vi "contador.vi"() -> ()   [LabVIEW 2009]
panel:
  out "y":dbl
  out "?":u8
  out "decimal integer string":string
  out "floor(x/y)":i32
  out "array":dbl[][](array[numeric])
  out "Array":dbl[][][](array[numeric])
  out "data out":string
  in  "id":i32
  in  "buffer":i32=300
  in  "number data":i32=1
  out "adreça":i32
  in  "command":i32
  in  "stop":bool
  in  "Send":bool
  out "data logged":string
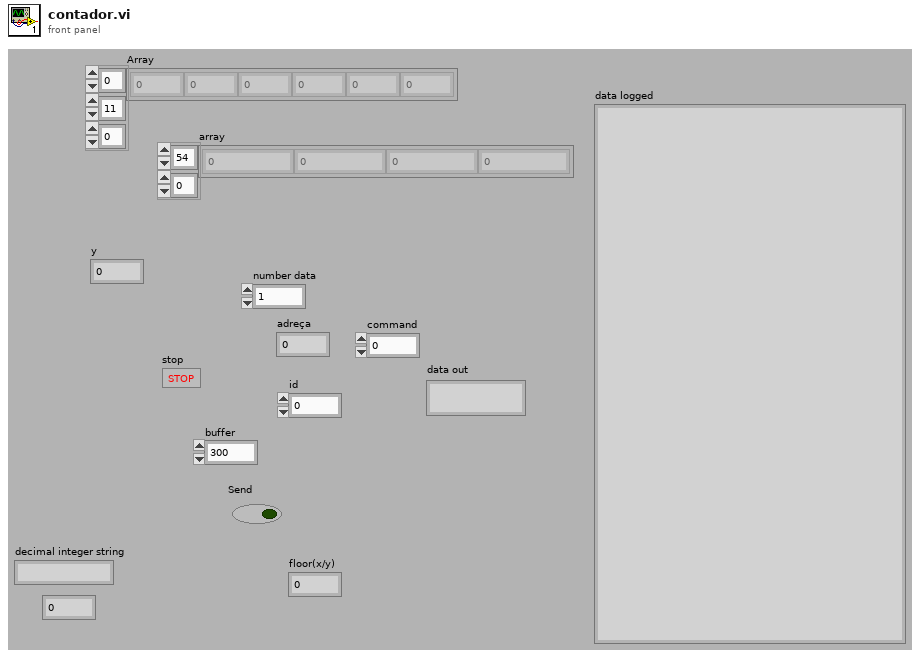
[diagram p1: front panel]
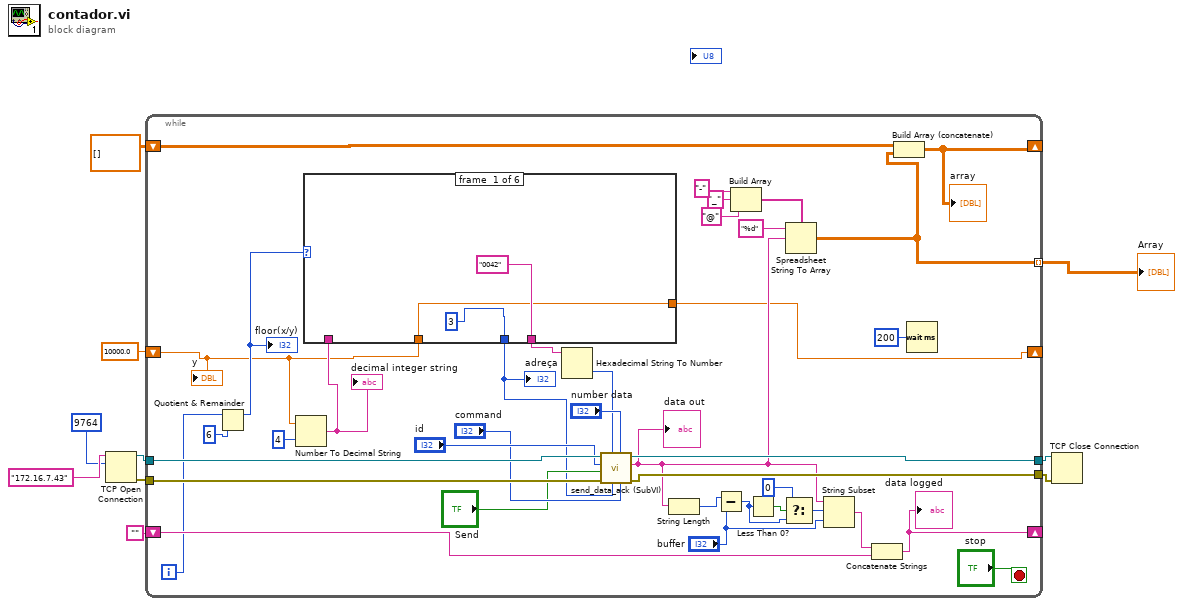
[diagram p0: block diagram]
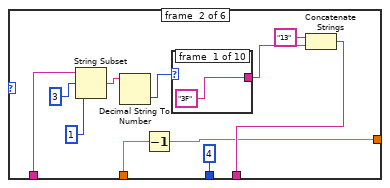
[diagram p2: hidden frame]
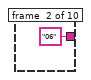
[diagram p3: hidden frame]
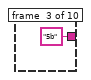
[diagram p4: hidden frame]
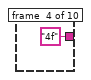
[diagram p5: hidden frame]
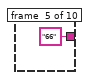
[diagram p6: hidden frame]
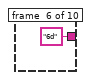
[diagram p7: hidden frame]
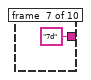
[diagram p8: hidden frame]
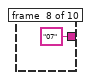
[diagram p9: hidden frame]
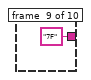
[diagram p10: hidden frame]
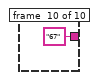
[diagram p11: hidden frame]
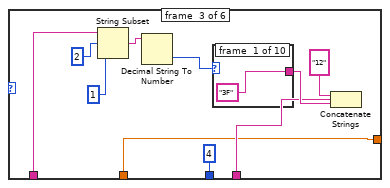
[diagram p12: hidden frame]
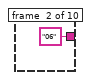
[diagram p13: hidden frame]
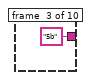
[diagram p14: hidden frame]
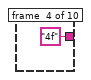
[diagram p15: hidden frame]
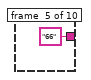
[diagram p16: hidden frame]
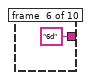
[diagram p17: hidden frame]
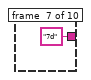
[diagram p18: hidden frame]
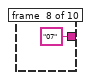
[diagram p19: hidden frame]
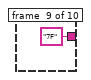
[diagram p20: hidden frame]
diagram:
  n1 = TCP Open Connection(address="172.16.7.43", remote port or service name=u16 9764) -> (connection ID=w5:refnum<k5>, error out=w4:errorcluster)  [unwired: 3 in]
  n2 = while {
    shift-right: [w40] -> _
    shift-left: "" -> [w39]
    tunnel: [w38] -> w9
    tunnel: [w37] -> w8
    tunnel: w5 -> [w36]
    tunnel: w4 -> [w35]
    tunnel: [w25] -> w3 mode=indexing
    shift-right: [w23] -> _
    shift-left: dbl[][] [] -> [w24]
    shift-right: [w12] -> _
    shift-left: 10000.0 ("y") -> [w11]
    i -> [w13]
    stop <- "stop" stop-if-true
    n3 = Quotient & Remainder(x=w13, y=6) -> (x-y*floor(x/y)=w16:i32)  [unwired: 1 out]
    "floor(x/y)" <- w16
    n4 = Number To Decimal String(number=w11, width (-)=i16 4) -> (decimal integer string=w14:string)
    "decimal integer string" <- w14
    n5 = case shown="3" w16 {
      tunnel: [3 ("adreça") 4 ("adreça") 4 ("adreça") 3 ("adreça") 4 ("adreça") 4 ("adreça")] -> w18
      tunnel: ["0042" ("string") w60 w79 "0040" ("string") w103 w122] -> w19
      tunnel: w14 -> [_ w58 w74 _ w97 w118]
      tunnel: w11 -> [w49 w53 w73 w93 w96 w116]
      tunnel: [w49 w52 w73 w93 w96 w116] -> w12
      frame #0 {
      }
      frame #1 {
        n6 = String Subset(string=w58, offset (0)=3 ("index"), length (rest)=1 ("length (rest)")) -> (substring=w55:string)
        n7 = Decimal String To Number(string=w55) -> (number=w54:i32)  [unwired: 2 in, 1 out]
        n8 = Decrement(x=w53) -> (x-1=w52:dbl)
        n9 = case shown="5" w54 {
          tunnel: ["3F" ("Data hex") "06" ("Data hex") "5b" ("Data hex") "4f" ("Data hex") "66" ("Data hex") "6d" ("Data hex") "7d" ("Data hex") "07" ("Data hex") "7F" ("Data hex") "67" ("Data hex")] -> w62
          frame #0 {
          }
          frame #1 {
          }
          frame #2 {
          }
          frame #3 {
          }
          frame #4 {
          }
          frame #5 {
          }
          frame #6 {
          }
          frame #7 {
          }
          frame #8 {
          }
          frame #9 {
          }
        }
        n10 = Concatenate Strings("13" ("string"), w62) -> (w60:string)
      }
      frame #2 {
        n11 = String Subset(string=w74, offset (0)=2 ("index"), length (rest)=1 ("length (rest)")) -> (substring=w76:string)
        n12 = Decimal String To Number(string=w76) -> (number=w75:i32)  [unwired: 2 in, 1 out]
        n13 = case shown="5" w75 {
          tunnel: ["3F" ("Data hex") "06" ("Data hex") "5b" ("Data hex") "4f" ("Data hex") "66" ("Data hex") "6d" ("Data hex") "7d" ("Data hex") "07" ("Data hex") "7F" ("Data hex") "67" ("Data hex")] -> w82
          frame #0 {
          }
          frame #1 {
          }
          frame #2 {
          }
          frame #3 {
          }
          frame #4 {
          }
          frame #5 {
          }
          frame #6 {
          }
          frame #7 {
          }
          frame #8 {
          }
          frame #9 {
          }
        }
        n14 = Concatenate Strings("12" ("string"), w82) -> (w79:string)
      }
      frame #3 {
      }
      frame #4 {
        n15 = String Subset(string=w97, offset (0)=1 ("index"), length (rest)=1 ("length (rest)")) -> (substring=w99:string)
        n16 = Decimal String To Number(string=w99) -> (number=w98:i32)  [unwired: 2 in, 1 out]
        n17 = case shown="9" w98 {
          tunnel: ["3F" ("Data hex") "06" ("Data hex") "5b" ("Data hex") "4f" ("Data hex") "66" ("Data hex") "6d" ("Data hex") "7d" ("Data hex") "07" ("Data hex") "7F" ("Data hex") "67" ("Data hex")] -> w105
          frame #0 {
          }
          frame #1 {
          }
          frame #2 {
          }
          frame #3 {
          }
          frame #4 {
          }
          frame #5 {
          }
          frame #6 {
          }
          frame #7 {
          }
          frame #8 {
          }
          frame #9 {
          }
        }
        n18 = Concatenate Strings("13" ("string"), w105) -> (w103:string)
      }
      frame #5 {
        n19 = String Subset(string=w118, offset (0)=0 ("index"), length (rest)=1 ("length (rest)")) -> (substring=w120:string)
        n20 = Decimal String To Number(string=w120) -> (number=w119:i32)  [unwired: 2 in, 1 out]
        n21 = case shown="5" w119 {
          tunnel: ["3F" ("Data hex") "06" ("Data hex") "5b" ("Data hex") "4f" ("Data hex") "66" ("Data hex") "6d" ("Data hex") "7d" ("Data hex") "07" ("Data hex") "7F" ("Data hex") "67" ("Data hex")] -> w125
          frame #0 {
          }
          frame #1 {
          }
          frame #2 {
          }
          frame #3 {
          }
          frame #4 {
          }
          frame #5 {
          }
          frame #6 {
          }
          frame #7 {
          }
          frame #8 {
          }
          frame #9 {
          }
        }
        n22 = Concatenate Strings("12" ("string"), w125) -> (w122:string)
      }
    }
    "adreça" <- w18
    n23 = Hexadecimal String To Number(string=w19) -> (number=w20:u32)  [unwired: 2 in, 1 out]
    n24 = call "send_data_ack (SubVI).vi"("command"="command", "number data"="number data", "adreça"=w18, "Dada"=w20, "error out"=w35, "Send"="Send", "id"="id", "connection ID"=w36) -> ("error out 2"=w37:errorcluster, "data out"=w31:string, "connection ID out"=w38:refnum<k5>)  [unwired: 1 out]
    "data out" <- w31
    n25 = String Length(string=w31) -> (length=w47:i32)
    n26 = Subtract(x=w47, y="buffer") -> (x-y=w44:i32)
    n27 = Build Array("-" ("spreadsheet string"), "_" ("element"), "@" ("element")) -> (w29:string[])
    n28 = Less Than 0?(x=w44) -> (x < 0?=w46:bool)
    n29 = Select(t=0, s=w46, f=w44) -> (s? t:f=w43:i32)
    n30 = Spreadsheet String To Array(delimiter (Tab)=w29, format string="%d", spreadsheet string=w31) -> (array=w25:dbl[][])  [unwired: 1 in]
    n31 = String Subset(string=w31, offset (0)=w43, length (rest)="buffer") -> (substring=w41:string)
    n32 = Concatenate Strings(w41, w39) -> (w40:string)
    "data logged" <- w40
    n33 = Build Array (concatenate)(w24, w25) -> (w23:dbl[][])
    "array" <- w23
    n34 = Wait (ms)(milliseconds to wait=u32 200) -> ()  [unwired: 1 out]
    "y" <- w11
  }
  "Array" <- w3
  n35 = TCP Close Connection(connection ID=w9, error in (no error)=w8) -> ()  [unwired: 1 in, 2 out]
